vi "Convert U16 to U8.vi"(0 "Image Src":T1, 2 "Max Value":i32=15, 5 "Image Dst":T1, 11 "Error in (no error)":errorcluster, 13 "Min Value":i32) -> (4 "Image Out":T1, 6 "Factor":dbl, 15 "Error out":errorcluster)   [LabVIEW 2021]
uses:
  <vilib>/vision/NI_Vision_Development_Module.lvlib
  <vilib>/vision/Image Controls.llb/IMAQ Image.ctl
panel:
  out "Original":T1(plugin-control)
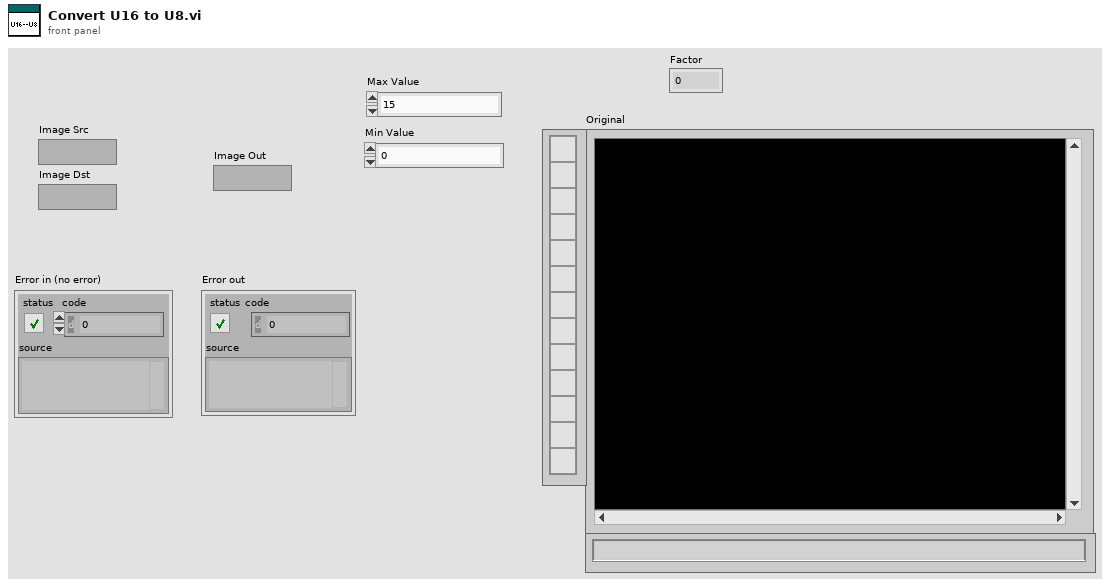
[diagram p1: front panel]
types:
  T1 = typedef "IMAQ Image.ctl" = refnum<image>
  T2 = typedef "Image Type" = u32
  T3 = cluster{"histogram":u32[], "Minimal Value":sgl, "Maximal Value":sgl, "Starting Value":sgl, "Interval Width":sgl, "Mean Value":sgl, "Standard  Variation":sgl, "Area (pixels)":i32}
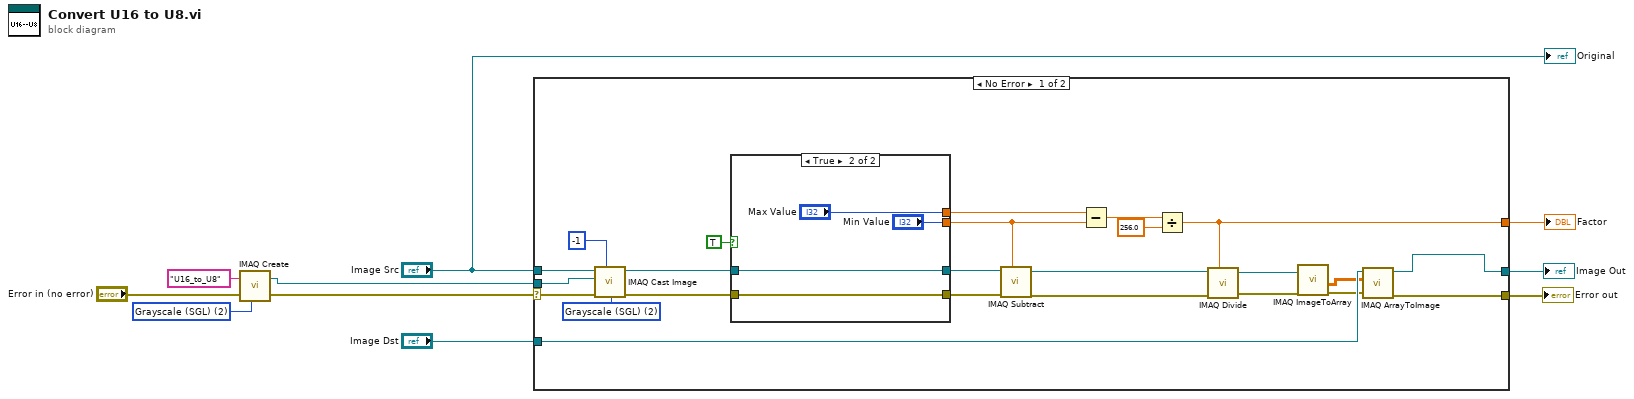
[diagram p0: block diagram]
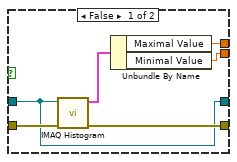
[diagram p2: hidden frame]
diagram:
  w4 = T2 2 items=["Grayscale (U8)", "Grayscale (I16)", "Grayscale (SGL)", "Complex (CSG)", "RGB (U32)", "HSL (U32)", "RGB (U64)", "Grayscale (U16)"] ("Image Type")
  n1 = call "IMAQ Create"("Image Name"="U16_to_U8", "Image Type"=w4, "error in (no error)"="Error in (no error)") -> ("New Image"=w3:T1, "error out"=w5:errorcluster)  [unwired: 2 in]
  n2 = case shown="No Error" w5 {
    selector: w5 -> [w25 w45]
    tunnel: [w14 w45] -> w10
    tunnel: "Image Src" -> [w29 _]
    tunnel: [w18 _] -> w9
    tunnel: "Image Dst" -> [w19 _]
    tunnel: [w21 _] -> w7
    tunnel: w3 -> [w12 _]
    frame No Error {
      w31 = T2 2 items=["Grayscale (U8)", "Grayscale (I16)", "Grayscale (SGL)", "Complex (CSG)", "RGB (U32)", "HSL (U32)", "RGB (U64)", "Grayscale (U16)"] ("Image Type")
      n3 = call "IMAQ Cast Image"("Image Type"=w31, "# Shifts"=-1, "error in (no error)"=w25, "Image Dst"=w12, "Image Src"=w29) -> ("error out"=w28:errorcluster, "Image Dst Out"=w26:T1)  [unwired: 5 in]
      n4 = case shown="True" TRUE {
        tunnel: w28 -> [w39 w44]
        tunnel: [w38 w44] -> w27
        tunnel: w26 -> [w37 w43]
        tunnel: [w37 w43] -> w24
        tunnel: [w36 "Max Value"] -> w23
        tunnel: [w35 "Min Value"] -> w22
        frame False {
          n5 = call "IMAQ Histogram"("error in (no error)"=w39, "Image"=w37) -> ("error out"=w38:errorcluster, "Histogram Report"=w40:T3)  [unwired: 8 in]
          n6 = Unbundle By Name(w40) -> ("Maximal Value"=w36:sgl, "Minimal Value"=w35:sgl)
        }
        frame True {
        }
      }
      n7 = call "IMAQ Subtract"("Image Src A"=w24, "Constant"=w22, "error in (no error)"=w27) -> ("Image Dst Out"=w32:T1, "error out"=w30:errorcluster)  [unwired: 4 in]
      n8 = Subtract(x=w23, y=w22) -> (x-y=w34:sgl)
      n9 = Divide(x=w34, y=256.0) -> (x/y=w21:dbl)
      n10 = call "IMAQ Divide"("Image Src A"=w32, "Constant"=w21, "error in (no error)"=w30) -> ("Image Dst Out"=w13:T1, "error out"=w17:errorcluster)  [unwired: 4 in]
      n11 = call "IMAQ ImageToArray"("error in (no error)"=w17, "Image"=w13) -> ("Image Pixels (Float)"=w15:sgl[][], "error out"=w16:errorcluster)  [unwired: 2 in, 3 out]
      n12 = call "IMAQ ArrayToImage"("error in (no error)"=w16, "Image Pixels (U8)"=w15, "Image"=w19) -> ("error out"=w14:errorcluster, "Image Out"=w18:T1)  [unwired: 7 in]
    }
    frame Error {
    }
  }
  "Error out" <- w10
  "Image Out" <- w9
  "Factor" <- w7
  "Original" <- "Image Src"
